vi "LabVIEW Not Complex And Operations.vi"(11 "X size":i32=16384) -> (3 "LabVIEW Time":dbl)   [LabVIEW 2020]
uses:
  <vilib>/Analysis/NI_AALBase.lvlib
panel:
  in  "num_loop":i32=6
  out "max value 2":sgl
  out "max value":sgl
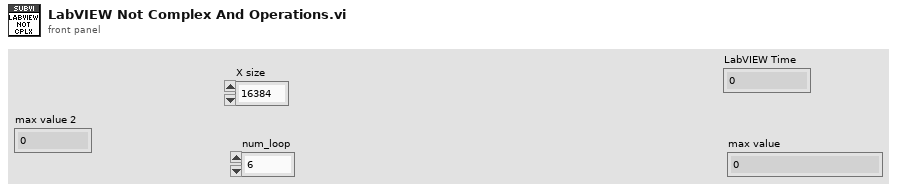
[diagram p1: front panel]
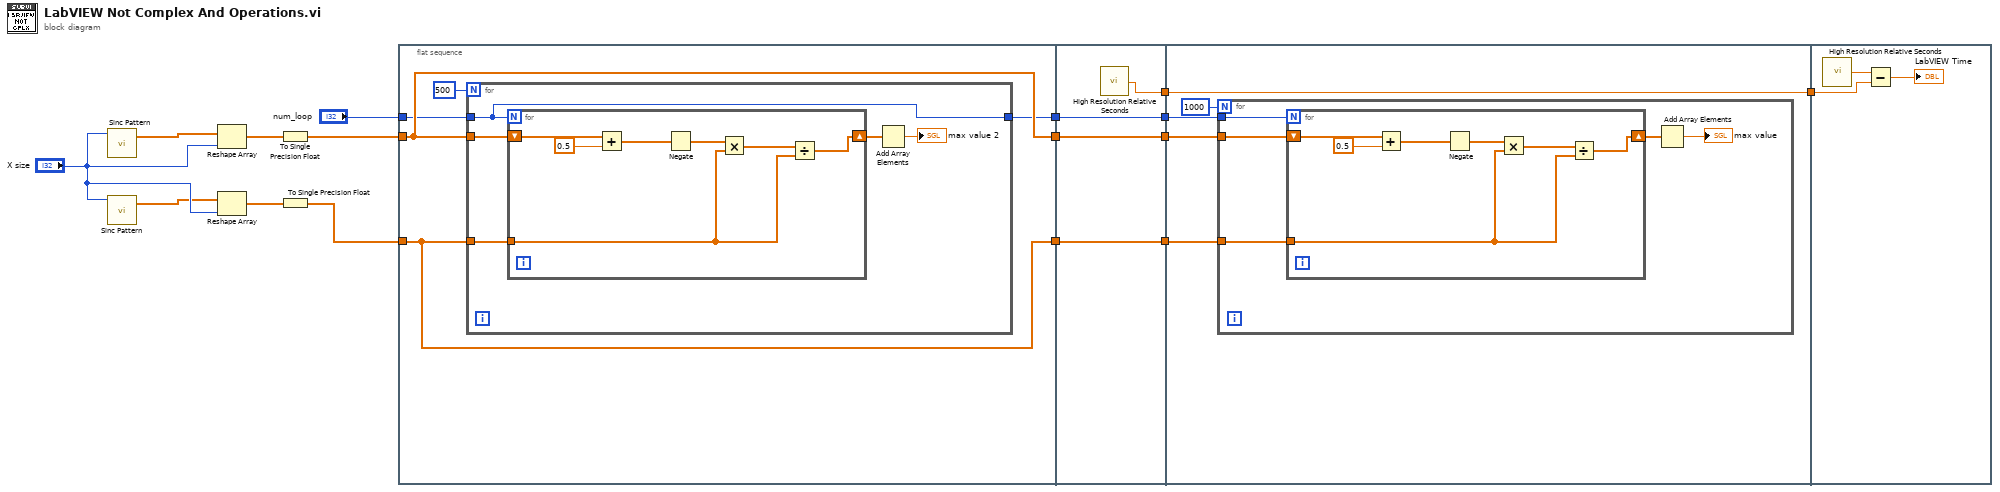
[diagram p0: block diagram]
diagram:
  n1 = call <vilib>:"Sinc Pattern.vi"("samples"="X size") -> ("Sinc Pattern"=w2:dbl[])  [unwired: 3 in, 1 out]
  n2 = call <vilib>:"Sinc Pattern.vi"("samples"="X size") -> ("Sinc Pattern"=w1:dbl[])  [unwired: 3 in, 1 out]
  n3 = Reshape Array(w2, "X size") -> (w9:dbl[])
  n4 = Reshape Array(w1, "X size") -> (w8:dbl[])
  n5 = To Single Precision Float(number=w9) -> (single precision float=w7:sgl[])
  n6 = To Single Precision Float(number=w8) -> (single precision float=w6:sgl[])
  n7 = flat-sequence {
    tunnel: w6 -> [w19]
    tunnel: w7 -> [w20]
    tunnel: [w20] -> w12
    tunnel: [w19] -> w11
    tunnel: "num_loop" -> [w18]
    tunnel: [w17] -> w3
    tunnel: [w37] -> w16
    tunnel: [w36] -> w14
    tunnel: [w35] -> w13
    tunnel: w12 -> [w36]
    tunnel: w11 -> [w35]
    tunnel: [w34] -> w4
    tunnel: w3 -> [w34]
    tunnel: w16 -> [w42]
    tunnel: [w42] -> w15
    tunnel: w14 -> [w41]
    tunnel: w13 -> [w40]
    tunnel: w4 -> [w38]
    tunnel: w15 -> [w56]
    frame #0 {
      n8 = for {
        N: 500 -> [_]
        tunnel: w20 -> [w26]
        tunnel: w19 -> [w25]
        tunnel: w18 -> [w22]
        tunnel: [w22] -> w17
        n9 = for {
          N: w22 -> [_]
          tunnel: w25 -> [w30]
          shift-right: [w28] -> w24
          shift-left: w26 -> [w31]
          n10 = Add(x=w31, y=sgl 0.5) -> (x+y=w27:sgl[])
          n11 = Negate(x=w27) -> (-x=w32:sgl[])
          n12 = Multiply(x=w32, y=w30) -> (x*y=w33:sgl[])
          n13 = Divide(x=w33, y=w30) -> (x/y=w28:sgl[])
        }
        n14 = Add Array Elements(numeric array=w24) -> (sum=→"max value 2":sgl)
      }
    }
    frame #1 {
      n15 = call <vilib>:"High Resolution Relative Seconds.vi"() -> ("relative seconds"=w37:dbl)
    }
    frame #2 {
      n16 = for {
        N: 1000 -> [_]
        tunnel: w41 -> [w46]
        tunnel: w40 -> [w45]
        tunnel: w38 -> [w43]
        n17 = for {
          N: w43 -> [_]
          tunnel: w45 -> [w51]
          shift-right: [w49] -> w47
          shift-left: w46 -> [w52]
          n18 = Add(x=w52, y=sgl 0.5) -> (x+y=w48:sgl[])
          n19 = Negate(x=w48) -> (-x=w53:sgl[])
          n20 = Multiply(x=w53, y=w51) -> (x*y=w54:sgl[])
          n21 = Divide(x=w54, y=w51) -> (x/y=w49:sgl[])
        }
        n22 = Add Array Elements(numeric array=w47) -> (sum=→"max value":sgl)
      }
    }
    frame #3 {
      n23 = call <vilib>:"High Resolution Relative Seconds.vi"() -> ("relative seconds"=w57:dbl)
      n24 = Subtract(x=w57, y=w56) -> (x-y=→"LabVIEW Time":dbl)
    }
  }
